vi "频率测量_高频.vi"() -> ()   [LabVIEW 2013]
doc: "This example demonstrates how to count the pulse's edges."
uses:
  <userlib>/ArtDAQ/_SubVI/ArtDAQ_CreateCIFreqChan.vi
  <userlib>/ArtDAQ/_SubVI/ArtDAQ_CfgSampClkTiming.vi
  <userlib>/ArtDAQ/_SubVI/ArtDAQ_Read Counter DBL NSamp.vi
panel:
  in  "开始边沿":i32(ring)=10280 items=["上升"=10280, "下降"=10171]
  in  "测量时间":dbl=0.01 format="%#_13g"
  in  "每通道点数":i32=10
  in  "采样速率":dbl=10000.0 format="%#_13g"
  in  "有效边沿":i32(ring)=10280 items=["上升"=10280, "下降"=10171]
  in  "时钟源":string="/Dev1/PFI0"
  out "数据":dbl[](array[numeric])
  in  "计数器":string="Dev1/ctr0"
  in  "最小值":dbl=1e-06 format="%0.6f"
  in  "最大值":dbl=2000000.0 format="%0.6f"
  in  "Stop":bool
  out "错误输出":errorcluster
  # "通道属性"
  # "定时"
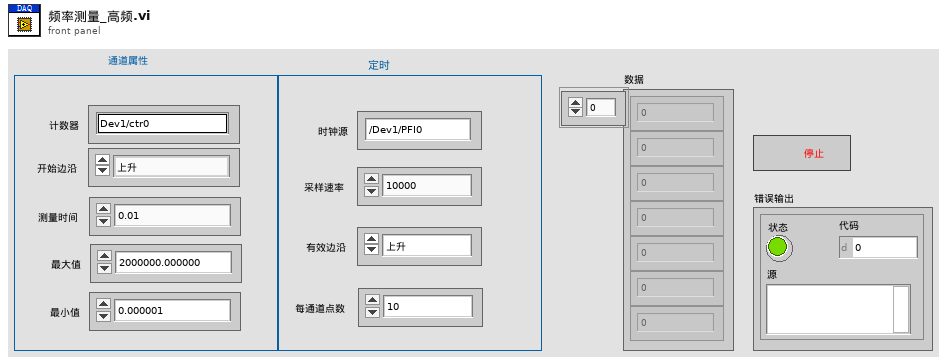
[diagram p1: front panel]
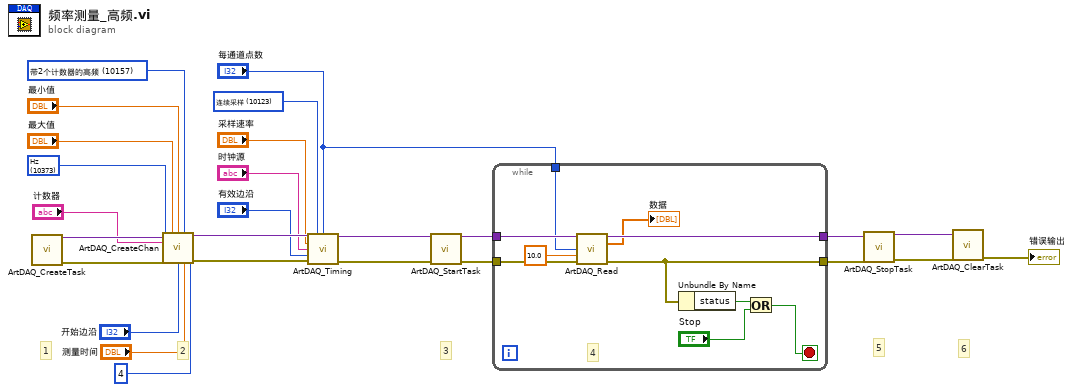
[diagram p0: block diagram]
diagram:
  w8 = 10157 items=["带1个计数器的低频"=10105, "带2个计数器的高频"=10157, "带2个计数器的大范围"=10205] ("测量方法")
  w9 = 10373 items=["Hz"=10373, "时钟滴答"=10304, "来自自定义换算"=10065] ("Units")
  w10 = 10123 items=["有限点采样"=10178, "连续采样"=10123] ("采样模式")
  # "6"
  # "5"
  # "3"
  # "2"
  # "1"
  n1 = call <userlib>:"ArtDAQ_CreateTask.vi"() -> ("任务句柄"=w26:variant, "错误输出"=w25:errorcluster)  [unwired: 14 in]
  n2 = call-poly <userlib>:"ArtDAQ_CreateChan.vi"("任务句柄"=w26, "最大值"="最大值", "最小值"="最小值", "测量方法"=w8, "计数器"="计数器", "除数"=u32 4 ("Divisor"), "单位"=w9, "错误输入"=w25, "开始边沿"="开始边沿", "测量时间"="测量时间") -> ("任务句柄"=w14:variant, "错误输出"=w11:errorcluster)  [unwired: 4 in]
  n3 = call-poly <userlib>:"ArtDAQ_Timing.vi"("任务句柄"=w14, "采样模式"=w10, "每通道采样数"="每通道点数", "采样率"="采样速率", "源"="时钟源", "有效边沿"="有效边沿", "错误输入"=w11) -> ("任务句柄"=w13:variant, "错误输出"=w12:errorcluster)  [unwired: 7 in]
  n4 = call <userlib>:"ArtDAQ_StartTask.vi"("任务句柄"=w13, "错误输入"=w12) -> ("任务句柄"=w18:variant, "错误输出"=w17:errorcluster)  [unwired: 12 in]
  n5 = while {
    tunnel: [w36] -> w23
    tunnel: [w35] -> w21
    tunnel: w18 -> [w34]
    tunnel: w17 -> [w33]
    tunnel: "每通道点数" -> [w29]
    stop <- w27 stop-if-true
    # "4"
    n6 = call-poly <userlib>:"ArtDAQ_Read.vi"("任务句柄"=w34, "每通道采样数"=w29, "超时s"=10.0 ("Timeout"), "错误输入"=w33) -> ("任务句柄"=w36:variant, "数据"=→"数据":dbl[], "错误输出"=w35:errorcluster)  [unwired: 8 in, 1 out]
    n7 = Unbundle By Name(w35) -> ("status"=w32:bool)
    n8 = Or(x=w32, y="Stop") -> (x .or. y?=w27:bool)
  }
  n9 = call <userlib>:"ArtDAQ_StopTask.vi"("任务句柄"=w23, "错误输入"=w21) -> ("任务句柄"=w22:variant, "错误输出"=w20:errorcluster)  [unwired: 12 in]
  n10 = call <userlib>:"ArtDAQ_ClearTask.vi"("任务句柄"=w22, "错误输入"=w20) -> ("错误输出"=→"错误输出":errorcluster)  [unwired: 13 in]
